vi "write password.vi"(8 "error in":errorcluster, 10 "password":string, 11 "syscfg device in":refnum<class "SysCfg Device.lvclass">) -> (0 "error out":errorcluster, 3 "syscfg device out":refnum<class "SysCfg Device.lvclass">)   [LabVIEW 2014, in "SMI.lvlib" / "SysCfg Device.lvclass"]
uses:
  SysCfg Device.lvclass
  SysCfg Device.lvclass/SysCfg Device.ctl
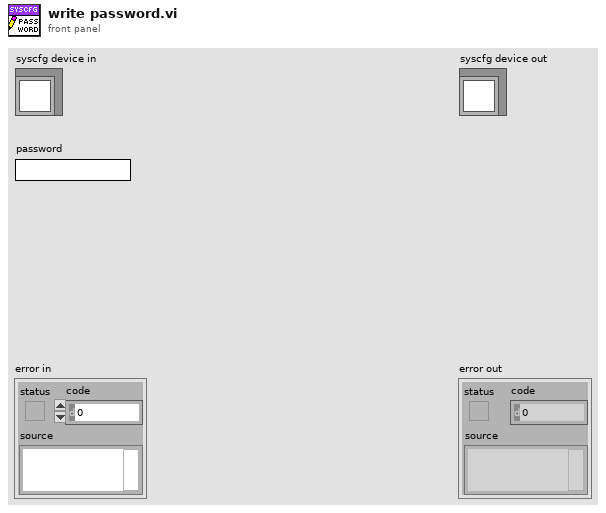
[diagram p1: front panel]
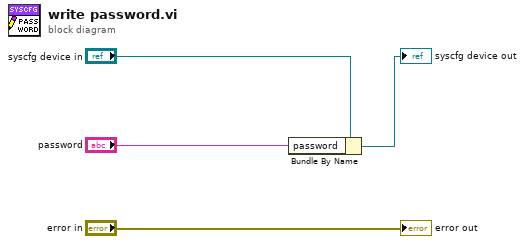
[diagram p0: block diagram]
diagram:
  n1 = Bundle By Name(cluster="syscfg device in", "password"="password") -> (→"syscfg device out":refnum<class "SysCfg Device.lvclass">)
  "error out" <- "error in"
